vi "Movement step (SILAR).vi"(6 "ENABLE контакт":u8, 7 "Шаговый двигатель №":u8, 8 "Error In":errorcluster, 9 "Скорость":i16=100, 10 "Кол-во шагов":i16, 11 "Arduino Resource In":T1={"VISA resource"="", "Board Type"=enum."Uno", "Connection Type"=enum."USB / Serial", "Bytes Per Packet (15)"=15}) -> (0 "Error Out":errorcluster, 3 "Arduino Resource Out":T1={"VISA resource"="", "Board Type"=enum."Uno", "Connection Type"=enum."USB / Serial", "Bytes Per Packet (15)"=15})   [LabVIEW 2016]
uses:
  <vilib>/LabVIEW Interface for Arduino/Type Defs/Arduino Resource.ctl
  <vilib>/LabVIEW Interface for Arduino/Type Defs/Board Type.ctl
  <vilib>/LabVIEW Interface for Arduino/LabVIEW Interface for Arduino.lvlib
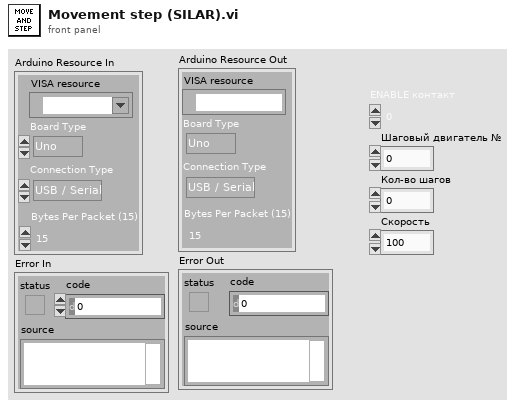
[diagram p1: front panel]
types:
  T1 = typedef "LabVIEW Interface for Arduino.lvlib/Arduino Resource.ctl" = cluster{"VISA resource":refnum<visa-resource-name>, "Board Type":T2, "Connection Type":enum8{"USB / Serial"}, "Bytes Per Packet (15)":u8}
  T2 = typedef "LabVIEW Interface for Arduino.lvlib/Board Type.ctl" = enum16{"Uno", "Dimuelanove w/Atmega 328", "Mega 2560"}
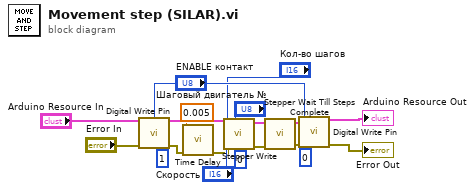
[diagram p0: block diagram]
diagram:
  n1 = call <vilib>:"Digital Write Pin.vi"("Arduino Resource"="Arduino Resource In", "Digital I/O Pin (0)"="ENABLE контакт", "Value (0)"=u8 1, "error in"="Error In") -> ("Arduino Resource"=w19:T1, "error out"=w5:errorcluster)  [unwired: 10 in]
  n2 = call "Time Delay"("error in (no error)"=w5, "Delay Time (s)"=0.005) -> ("error out"=w4:errorcluster)  [unwired: 9 in]
  n3 = call <vilib>:"Stepper Write.vi"("Set Acceleration (0 to disable)"=i16 0, "Stepper #"="Шаговый двигатель №", "error in"=w4, "Set Speed (Steps per Second)"="Скорость", "# of Steps to Move"="Кол-во шагов", "Arduino Resource"=w19) -> ("error out"=w16:errorcluster, "Arduino Resource Out"=w15:T1)  [unwired: 4 in]
  n4 = call <vilib>:"Stepper Wait Till Steps Complete.vi"("error in"=w16, "Arduino Resource In"=w15) -> ("error out"=w17:errorcluster, "Arduino Resource Out"=w18:T1)  [unwired: 8 in]
  n5 = call <vilib>:"Digital Write Pin.vi"("Arduino Resource"=w18, "Digital I/O Pin (0)"="ENABLE контакт", "Value (0)"=u8 0, "error in"=w17) -> ("Arduino Resource"=→"Arduino Resource Out":T1, "error out"=→"Error Out":errorcluster)  [unwired: 10 in]
